vi "ProcessJSONRunning.vi"(8 "error in (no error)":errorcluster, 11 "JSON Array":string) -> (0 "error out":errorcluster, 2 "JSON Error string":string, 3 "JSON Response String":string)   [LabVIEW 2013]
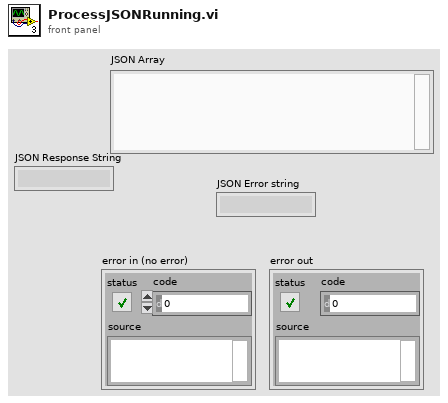
[diagram p1: front panel]
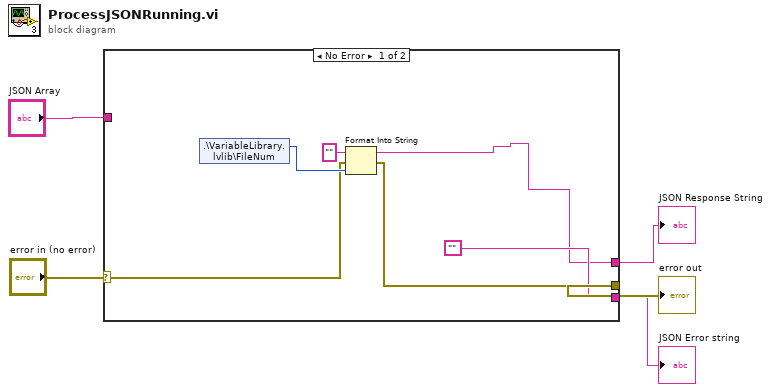
[diagram p0: block diagram]
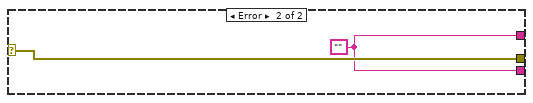
[diagram p2: hidden frame]
diagram:
  n1 = case shown="No Error" "error in (no error)" {
    selector: "error in (no error)" -> [w7 w13]
    tunnel: "JSON Array" -> [_ _]
    tunnel: [w6 w13] -> w5
    tunnel: ["" w12] -> w3
    tunnel: [w9 w12] -> w2
    frame No Error {
      n2 = shared-variable ".\\VariableLibrary.lvlib\\FileNum"() -> (w10:u32)  [unwired: 1 in, 1 out]
      n3 = Format Into String(initial string="", error in=w7, w10) -> (resulting string=w9:string, error out=w6:errorcluster)  [unwired: 1 in]
    }
    frame Error {
      w12 = ""
    }
  }
  "error out" <- w5
  "JSON Error string" <- w3
  "JSON Response String" <- w2
